vi "FP_to_DSC.vi"(8 "error in (no error)":errorcluster, 11 "FP cluster":T1) -> (0 "error IO":errorcluster)   [LabVIEW 2016]
uses:
  Typedefs/FP-cluster.ctl
  <vilib>/Platform/browser.llb/Open URL in Default Browser (string).vi
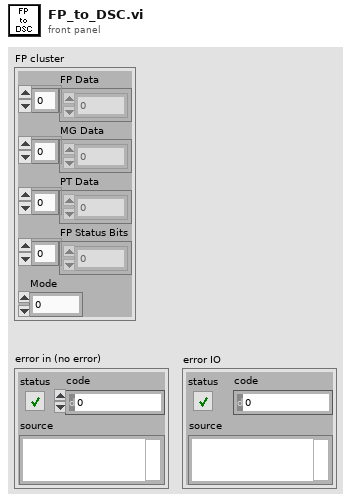
[diagram p1: front panel]
types:
  T1 = typedef "FP-cluster.ctl" = cluster{"FP Data":sgl[], "MG Data":dbl[], "PT Data":dbl[], "FP Status Bits":u32[], "Mode":u16}
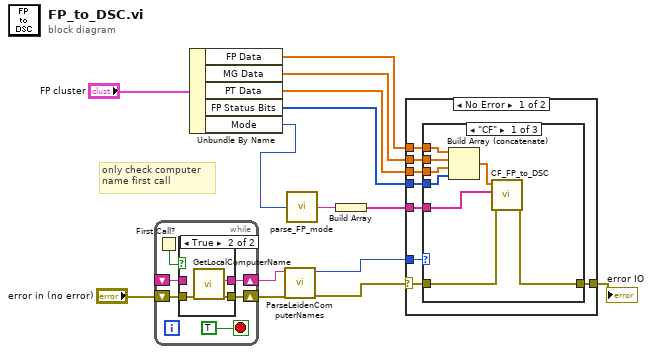
[diagram p0: block diagram]
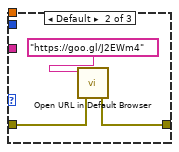
[diagram p3: hidden frame]
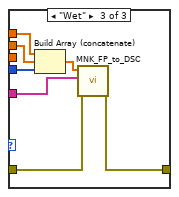
[diagram p4: hidden frame]
diagram:
  # "only check computer\nname first call"
  n1 = while {
    shift-right: [w19] -> w9
    shift-left: "error in (no error)" -> [w18]
    shift-right: [w20] -> w11
    shift-left: _ -> [w16]
    stop <- TRUE stop-if-true
    n2 = First Call?() -> (First Call?: T/F=w17:bool)
    n3 = case shown="True" w17 {
      tunnel: [w22 w25] -> w20
      tunnel: [w21 w24] -> w19
      tunnel: w18 -> [w21 w23]
      tunnel: w16 -> [w22 _]
      frame False {
      }
      frame True {
        n4 = call "GetLocalComputerName.vi"("error in (no error)"=w23) -> ("error out"=w24:errorcluster, "Name"=w25:string)  [unwired: 8 in, 1 out]
      }
    }
  }
  n5 = Unbundle By Name("FP cluster") -> ("FP Data"=w6:sgl[], "MG Data"=w5:dbl[], "PT Data"=w4:dbl[], "FP Status Bits"=w3:u32[], "Mode"=w1:u16)
  n6 = call "ParseLeidenComputerNames.vi"("error in (no error)"=w9, "computer name"=w11) -> ("error out"=w10:errorcluster, "FP Type"=w12:enum32{"CF", "Wet"})  [unwired: 7 in, 1 out]
  n7 = call "parse_FP_mode.vi"("line index"=w1) -> ("output string"=w13:string)
  n8 = Build Array(w13) -> (w14:string[])
  n9 = case shown="No Error" w10 {
    selector: w10 -> [w27 w52]
    tunnel: w14 -> [w33 _]
    tunnel: w4 -> [w32 _]
    tunnel: w5 -> [w31 _]
    tunnel: w6 -> [w30 _]
    tunnel: w3 -> [w29 _]
    tunnel: w12 -> [w28 _]
    tunnel: [w26 w52] -> w8
    frame No Error {
      n10 = case shown="\"CF\"" w28 {
        tunnel: w30 -> [w40 _ w51]
        tunnel: w31 -> [w39 _ w50]
        tunnel: w32 -> [w38 _ _]
        tunnel: w33 -> [w37 _ w47]
        tunnel: w29 -> [w36 _ w49]
        tunnel: w27 -> [w35 w43 w46]
        tunnel: [w34 w42 w45] -> w26
        frame "CF" {
          n11 = Build Array (concatenate)(w40, w39, w38, w36) -> (w41:dbl[])
          n12 = call "CF_FP_to_DSC.vi"("error in (no error)"=w35, "str"=w37, "dbl"=w41) -> ("error out"=w34:errorcluster)  [unwired: 8 in]
        }
        frame Default {
          n13 = call-poly <vilib>:"Open URL in Default Browser.vi"("error in (no error)"=w43, "URL"="https://goo.gl/J2EWm4") -> ("error out"=w42:errorcluster)  [unwired: 4 in, 1 out]
        }
        frame "Wet" {
          n14 = Build Array (concatenate)(w51, w50, w49) -> (w48:dbl[])
          n15 = call "MNK_FP_to_DSC.vi"("error in (no error)"=w46, "str"=w47, "dbl"=w48) -> ("error out"=w45:errorcluster)  [unwired: 8 in]
        }
      }
    }
    frame Error {
    }
  }
  "error IO" <- w8
